vi "Find LVClasses in lvlib.vi"(8 "error in (no error)":errorcluster, 11 "Library Path":path) -> (0 "error out":errorcluster, 2 "Class paths":path[](array[path]), 3 "Classes in library":string[](array[string]))   [LabVIEW 2020, in "Test Finder.lvclass"]
uses:
  Test Finder.lvclass
  Test Case/LUnit Test Case.lvclass
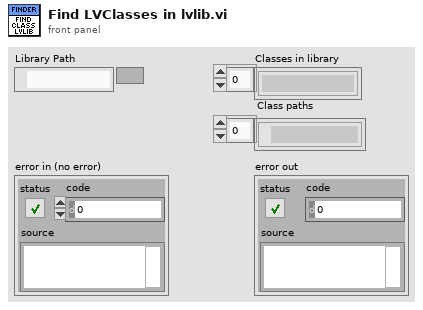
[diagram p1: front panel]
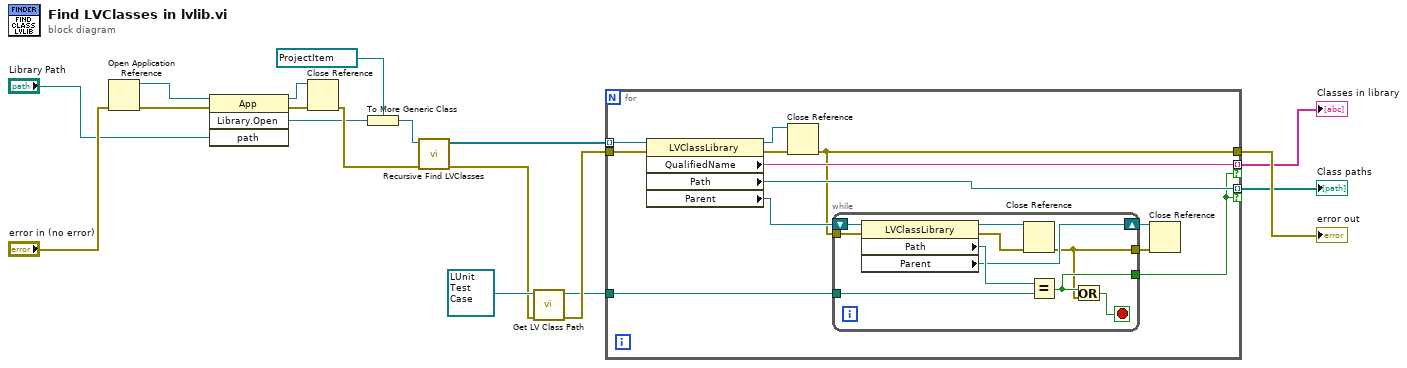
[diagram p0: block diagram]
diagram:
  n1 = Open Application Reference(8:"error in (no error)") -> (0:w11:errorcluster, 3:w10:refnum<vi>)  [unwired: 3 in]
  n2 = invoke class="App" method="Library.Open"(reference=w10, error in=w11, "path"="Library Path") -> (reference out=w13:refnum<vi>, error out=w12:errorcluster, "Open Library"=w6:refnum<vi>)  [unwired: 1 in, 1 out]
  n3 = Close Reference(reference=w13, error in (no error)=w12) -> (error out=w18:errorcluster)
  n4 = To More Generic Class(target class=refnum<vi> refnum ("reference"), reference=w6) -> (generic class reference=w5:refnum<vi>)
  n5 = call "Recursive Find LVClasses.vi"("error in (no error)"=w18, "reference"=w5) -> ("error out"=w3:errorcluster, "Class References"=w14:refnum<vi>[])  [unwired: 8 in]
  n6 = call <vilib>:"Get LV Class Path.vi"("error in (no error)"=w3, "object"=refnum<class "LUnit Test Case.lvclass"> refnum ("LUnit Test Case.lvclass")) -> ("error out"=w2:errorcluster, "class path"=w1:path)  [unwired: 8 in]
  n7 = for {
    tunnel: w14 -> [w30] mode=indexing
    tunnel: w2 -> [w29]
    tunnel: [w28] -> w15 mode=indexing if=w21
    tunnel: [w23] -> w17
    tunnel: [w25] -> w8 mode=indexing if=w21
    tunnel: w1 -> [w22]
    n8 = property class="LVClassLibrary"(reference=w30, error in=w29) -> (reference out=w26:refnum<vi>, error out=w27:errorcluster, "QualifiedName"=w28:string, "Path"=w25:path, "Parent"=w24:refnum<vi>)
    n9 = Close Reference(reference=w26, error in (no error)=w27) -> (error out=w23:errorcluster)
    n10 = while {
      tunnel: w23 -> [w39]
      tunnel: w22 -> [w35]
      tunnel: [w33] -> w21
      shift-right: [w32] -> w19
      shift-left: w24 -> [w40]
      tunnel: [w31] -> w20
      stop <- w34 stop-if-true
      n11 = property class="LVClassLibrary"(reference=w40, error in=w39) -> (reference out=w37:refnum<vi>, error out=w38:errorcluster, "Path"=w36:path, "Parent"=w32:refnum<vi>)
      n12 = Close Reference(reference=w37, error in (no error)=w38) -> (error out=w31:errorcluster)
      n13 = Equal?(x=w36, y=w35) -> (x = y?=w33:bool)
      n14 = Or(x=w33, y=w31) -> (x .or. y?=w34:bool)
    }
    n15 = Close Reference(reference=w19, error in (no error)=w20) -> ()  [unwired: 1 out]
  }
  "error out" <- w17
  "Classes in library" <- w15
  "Class paths" <- w8
